vi "InitCalibrationState.vi"   [LabVIEW 2013]
uses:
  GlobalVariables/CalibrationState.vi
types:
  T1 = cluster{bool, "CalibrationState":u32, "Volumes":dbl[], "PressureRatios":dbl[]}
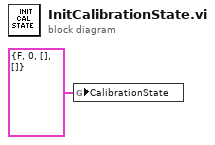
[diagram p0: block diagram]
diagram:
  n1 = global write "CalibrationState.vi" "CalibrationState"(T1 {FALSE, "CalibrationState"=0, "Volumes"=[], "PressureRatios"=[]} ("CalibrationState")) -> ()
